vi "mini_AC_read_data.vi"() -> ()   [LabVIEW 2016]
uses:
  <vilib>/Analysis/6fits.llb/Curve Fitting Criteria.ctl
  <vilib>/Instr/_visa.llb/VISA Configure Serial Port (Instr).vi
  <vilib>/Utility/file.llb/Write Delimited Spreadsheet (DBL).vi
  <vilib>/Analysis/NI_AALPro.lvlib
panel:
  out "Tau / fs":dbl
  out "standard deviation":dbl format="%#_3g"
  in  "Save path":path=path "E:/data/ProPlasMod/2023_02_24_DELL"
  in  "VISA resource name":refnum<visa-resource-name>="COM8"
  out "XY Graph":T1(graph)
  in  "Serial Settings:Baud Rate":u32=38400
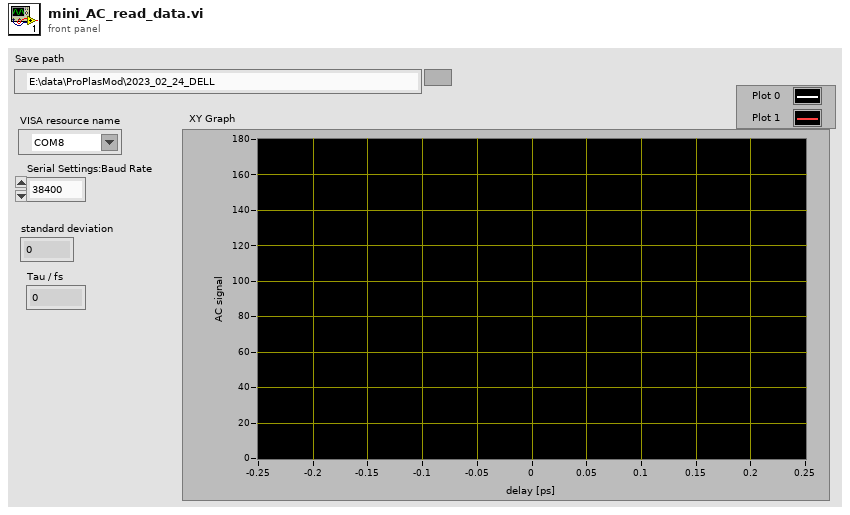
[diagram p1: front panel]
types:
  T1 = cluster{"array out":dbl[], "Best Gaussian Fit":dbl[]}[]
  T2 = cluster{"amp min":dbl, "amp max":dbl, "center min":dbl, "center max":dbl, "deviation min":dbl, "deviation max":dbl, "offset min":dbl, "offset max":dbl}
  T3 = typedef "NI_AALPro.lvlib/Curve Fitting Criteria.ctl" = u16
  T4 = cluster{"array out":dbl[], "unsigned byte array":u8[]}
  T5 = cluster{"array out":dbl[], "Best Gaussian Fit":dbl[]}
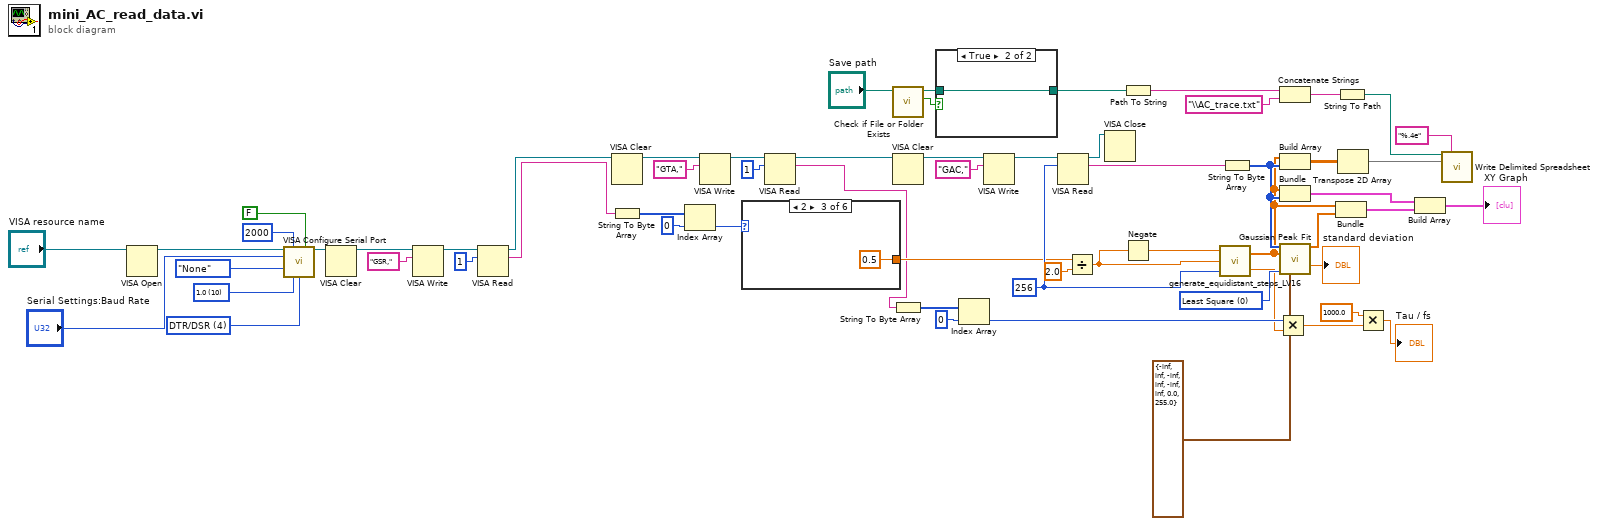
[diagram p0: block diagram]
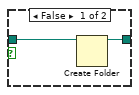
[diagram p2: hidden frame]
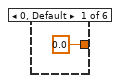
[diagram p3: hidden frame]
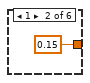
[diagram p4: hidden frame]
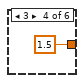
[diagram p5: hidden frame]
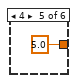
[diagram p6: hidden frame]
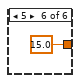
[diagram p7: hidden frame]
diagram:
  w10 = u16 10 items=["1.0"=10, "1.5"=15, "2.0"=20] ("stop bits (10: 1 bit)")
  w28 = T3 0 items=["Least Square", "Least Absolute Residual", "Bisquare"] ("method")
  w45 = u32 256 ("byte count")
  w58 = u16 4 items=["None", "XON/XOFF", "RTS/CTS", "XON/XOFF & RTS/CTS", "DTR/DSR", "XON/XOFF & DTR/DSR"] ("flow control (0:none)")
  n1 = VISA Open(VISA resource name="VISA resource name") -> (VISA resource name=w60:refnum<visa-resource-name>)  [unwired: 4 in, 1 out]
  n2 = call-poly "VISA Configure Serial Port"("VISA resource name"=w60, "timeout (10sec)"=u32 2000, "Enable Termination\nChar (T)"=FALSE ("Enable Termination\nChar (T)"), "baud rate (9600)"="Serial Settings:Baud Rate", "parity (0:none)"=enum16{"None", "Odd", "Even", "Mark", "Space"}."None", "stop bits (10: 1 bit)"=w10, "flow control (0:none)"=w58) -> ("VISA resource name out"=w56:refnum<visa-resource-name>)  [unwired: 7 in, 1 out]
  n3 = VISA Clear(VISA resource name=w56) -> (VISA resource name out=w4:refnum<visa-resource-name>)  [unwired: 1 in, 1 out]
  n4 = VISA Write(VISA resource name=w4, write buffer="GSR,") -> (VISA resource name out=w51:refnum<visa-resource-name>)  [unwired: 1 in, 2 out]
  n5 = VISA Read(VISA resource name=w51, byte count=u32 1) -> (VISA resource name out=w8:refnum<visa-resource-name>, read buffer=w49:string)  [unwired: 1 in, 2 out]
  n6 = VISA Clear(VISA resource name=w8) -> (VISA resource name out=w5:refnum<visa-resource-name>)  [unwired: 1 in, 1 out]
  n7 = String To Byte Array(string=w49) -> (unsigned byte array=w48:u8[])
  n8 = Index Array(array=w48, index=0) -> (element=w46:u8)
  n9 = VISA Write(VISA resource name=w5, write buffer="GTA,") -> (VISA resource name out=w3:refnum<visa-resource-name>)  [unwired: 1 in, 2 out]
  n10 = case shown="2" w46 {
    tunnel: [0.0 0.15 0.5 1.5 5.0 15.0] -> w44
    frame 0, Default {
    }
    frame 1 {
    }
    frame 2 {
    }
    frame 3 {
    }
    frame 4 {
    }
    frame 5 {
    }
  }
  n11 = VISA Read(VISA resource name=w3, byte count=u32 1) -> (VISA resource name out=w7:refnum<visa-resource-name>, read buffer=w17:string)  [unwired: 1 in, 2 out]
  n12 = call <vilib>:"Check if File or Folder Exists.vi"("path"="Save path") -> ("file or folder exists?"=w39:bool, "dup path"=w38:path)  [unwired: 8 in, 1 out]
  n13 = VISA Clear(VISA resource name=w7) -> (VISA resource name out=w2:refnum<visa-resource-name>)  [unwired: 1 in, 1 out]
  n14 = String To Byte Array(string=w17) -> (unsigned byte array=w19:u8[])
  n15 = case shown="True" w39 {
    tunnel: [w68 w70] -> w37
    tunnel: w38 -> [w69 w70]
    frame False {
      n16 = Create Folder(path (use dialog)=w69) -> (created path=w68:path)  [unwired: 2 in, 2 out]
    }
    frame True {
    }
  }
  n17 = Index Array(array=w19, index=0) -> (element=w16:u8)
  n18 = VISA Write(VISA resource name=w2, write buffer="GAC,") -> (VISA resource name out=w52:refnum<visa-resource-name>)  [unwired: 1 in, 2 out]
  n19 = VISA Read(VISA resource name=w52, byte count=w45) -> (VISA resource name out=w6:refnum<visa-resource-name>, read buffer=w54:string)  [unwired: 1 in, 2 out]
  n20 = Divide(x=w44, y=2.0) -> (x/y=w41:dbl)
  n21 = VISA Close(VISA resource name=w6) -> ()  [unwired: 1 in, 1 out]
  n22 = Path To String(path=w37) -> (string=w35:string)
  n23 = Negate(x=w41) -> (-x=w42:dbl)
  n24 = call "generate_equidistant_steps_LV16.vi"("# of steps"=w45, "end value"=w41, "start value"=w42) -> ("stepsize"=w15:dbl, "array out"=w26:dbl[])
  n25 = String To Byte Array(string=w54) -> (unsigned byte array=w29:u8[])
  n26 = Multiply(x=w16, y=w15) -> (x*y=w14:dbl)
  n27 = Concatenate Strings(w35, "\\AC_trace.txt" ("string")) -> (w33:string)
  n28 = Build Array(w26, w29) -> (w31:dbl[][])
  n29 = Bundle("array out"=w26, "unsigned byte array"=w29) -> (w24:T4)  [unwired: 1 in]
  n30 = call <vilib>:"Gaussian Peak Fit.vi"("Y"=w29, "X"=w26, "method"=w28, "parameter bounds"=T2 {"amp min"=-inf, "amp max"=inf, "center min"=-inf, "center max"=inf, "deviation min"=-inf, "deviation max"=inf, "offset min"=0.0, "offset max"=255.0}) -> ("Best Gaussian Fit"=w25:dbl[], "standard deviation"=→"standard deviation":dbl)  [unwired: 5 in, 5 out]
  n31 = Bundle("array out"=w26, "Best Gaussian Fit"=w25) -> (w23:T5)  [unwired: 1 in]
  n32 = String To Path(string=w33) -> (path=w32:path)
  n33 = Transpose 2D Array(2D array=w31) -> (transposed array=w30:dbl[][])
  n34 = Multiply(x=1000.0, y=w14) -> (x*y=→"Tau / fs":dbl)
  n35 = Build Array(w24, w23) -> (→"XY Graph":T1)
  n36 = call-poly <vilib>:"Write Delimited Spreadsheet.vi"("file path (dialog if empty)"=w32, "format (%.3f)"="%.4e", "2D data"=w30) -> ()  [unwired: 11 in, 2 out]
